vi "simple_write_array.vi"(8 "error in (no error)":errorcluster, 9 "path":string, 10 "Array":dbl[](array[numeric]), 11 "lfield_logger in":refnum<class "lfield_logger.lvclass">) -> (0 "error out":errorcluster, 3 "lfield_logger out":refnum<class "lfield_logger.lvclass">)   [LabVIEW 2015, in "lfield_logger.lvclass"]
uses:
  lfield_logger.lvclass
  Data Logger Class/data_logger.lvclass
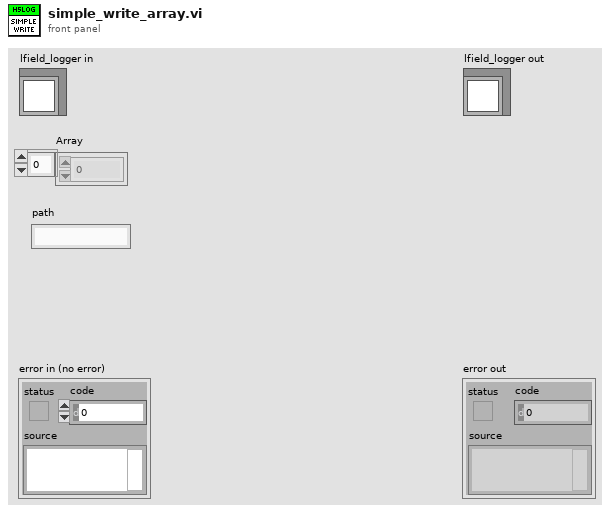
[diagram p1: front panel]
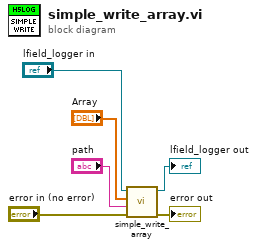
[diagram p0: block diagram]
diagram:
  n1 = call-parent "simple_write_array.vi"("error in (no error)"="error in (no error)", "path"="path", "Array"="Array", "data_logger in"="lfield_logger in") -> ("error out"=→"error out":errorcluster, "data_logger out"=→"lfield_logger out":refnum<class "lfield_logger.lvclass">)  [unwired: 6 in]
